vi "Stubs Dir.vi"() -> (3 "path":path)   [LabVIEW 2014, in "lvprj2html.lvlib"]
uses:
  lvprj2html.lvlib
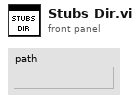
[diagram p1: front panel]
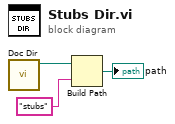
[diagram p0: block diagram]
diagram:
  n1 = call "Doc Dir.vi"() -> ("appended path"=w3:path)  [unwired: 10 in, 1 out]
  n2 = Build Path(base path=w3, name or relative path="stubs") -> (appended path=→"path":path)
